vi "Init GPIO Resources.vi"(8 "error in (no error)":errorcluster, 11 "Session in":refnum<class "Session.lvclass">) -> (0 "error out":errorcluster, 3 "Session out":refnum<class "Session.lvclass">)   [LabVIEW 2020, in "CTI.lvlib" / "Session.lvclass"]
uses:
  Session.lvclass
  GPIO Number.ctl
  GPIO/GPIO.lvclass
  Session.lvclass/Session.ctl
  DeviceComms/DeviceComms.lvclass
  CTI.lvlib
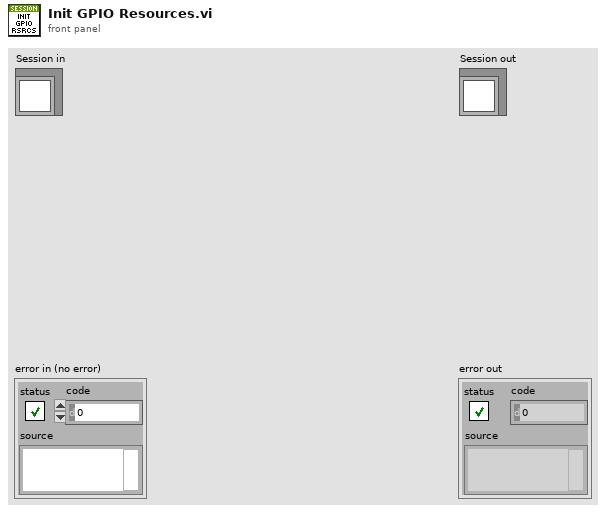
[diagram p1: front panel]
types:
  T1 = typedef "CTI.lvlib/GPIO Number.ctl" = i8
  T2 = typedef "CTI.lvlib/Session.lvclass/Resources.ctl" = cluster{"GPIO":map{T1, refnum<class "GPIO.lvclass">}, "AI":map{T3, refnum<class "AI.lvclass">}, "PWM":map{T1, refnum<class "PWM.lvclass">}, "UART":map{T4, refnum<class "UART.lvclass">}, "I2C":map{T5, refnum<class "I2C.lvclass">}, "SPI":map{T6, refnum<class "SPI.lvclass">}, "CS":map{T1, refnum<class "SPI CS.lvclass">}}
  T3 = typedef "CTI.lvlib/ADC Number.ctl" = i8
  T4 = typedef "CTI.lvlib/UART Number.ctl" = i8
  T5 = typedef "CTI.lvlib/I2C Number.ctl" = i8
  T6 = typedef "CTI.lvlib/SPI Number.ctl" = i8
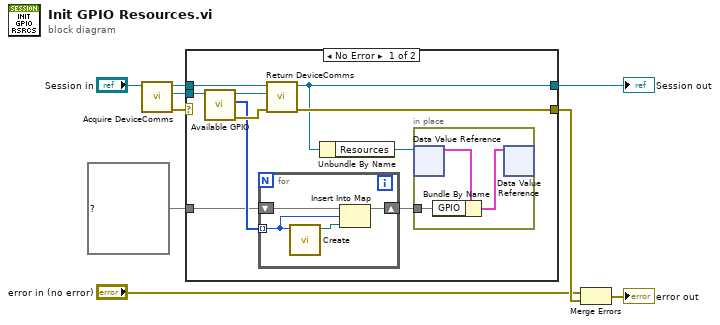
[diagram p0: block diagram]
diagram:
  n1 = call "Acquire DeviceComms.vi"("Session in"="Session in") -> ("error out"=w8:errorcluster, "DeviceComms"=w7:refnum<class "DeviceComms.lvclass">, "Session out"=w6:refnum<class "Session.lvclass">)  [unwired: 8 in]
  n2 = case shown="No Error" w8 {
    selector: w8 -> [_ w28]
    tunnel: w7 -> [w17 _]
    tunnel: w6 -> [w16 w27]
    tunnel: [w10 w27] -> w5
    tunnel: map{T1, refnum<class "GPIO.lvclass">} {} ("GPIO") -> [w13 _]
    tunnel: [w19 w28] -> w3
    frame No Error {
      n3 = call-dynamic "Available GPIO.vi"("DeviceComms in"=w17) -> ("error out"=w18:errorcluster, "Available GPIO"=w14:T1[], "DeviceComms out"=w15:refnum<class "DeviceComms.lvclass">)  [unwired: 8 in]
      n4 = for {
        tunnel: w14 -> [w25] mode=indexing
        shift-right: [w23] -> w11
        shift-left: w13 -> [w26]
        n5 = call "Create.vi"("GPIO #"=w25) -> ("GPIO out"=w24:refnum<class "GPIO.lvclass">)  [unwired: 9 in, 1 out]
        n6 = Insert Into Map(map in=w26, key=w25, value=w24) -> (map out=w23:map{T1, refnum<class "GPIO.lvclass">})  [unwired: 2 out]
      }
      n7 = call "Return DeviceComms.vi"("error in (no error)"=w18, "DeviceComms"=w15, "Session in"=w16) -> ("error out"=w19:errorcluster, "Session out"=w10:refnum<class "Session.lvclass">)  [unwired: 7 in]
      n8 = Unbundle By Name(w10) -> ("Resources"=w12:refnum<data-value>)
      n9 = in-place {
        in-place-border: w11 -> [w21]
        n10 = in-place-dvr #1(w12) -> (w22:T2)  [unwired: 1 out]
        n11 = Bundle By Name(cluster=w22, "GPIO"=w21) -> (w20:T2)
        n12 = in-place-dvr #1(w20) -> ()  [unwired: 2 out]
      }
    }
    frame Error {
    }
  }
  "Session out" <- w5
  n13 = Merge Errors("error in (no error)", w3) -> (→"error out":errorcluster)
